vi "retrieve.vi"(8 "error in (no error)":errorcluster, 11 "DL090215DataCollection in":refnum<class "DataCollectionDL090215.lvclass">) -> (0 "error out":errorcluster, 3 "DL090215DataCollection out":refnum<class "DataCollectionDL090215.lvclass">)   [LabVIEW 2010]
uses:
  DataRequest/GenericDataRequest/GenericDataRequest/GenericDataRequest.lvclass
  common/classes/ImageCollection/ImageCollection/ImageCollection.lvclass
  common/classes/Image/Image/Image.lvclass
  common/classes/Image/Image/storage_mode.ctl
  Display/GenericDisplay/GenericDisplay/GenericDisplay.lvclass
  common/classes/ImageCollection/ImageCollection/add_mode_enum.ctl
  common/classes/ErrorController/ErrorController/ErrorController.lvclass
  DataCollectionDL090215.lvclass
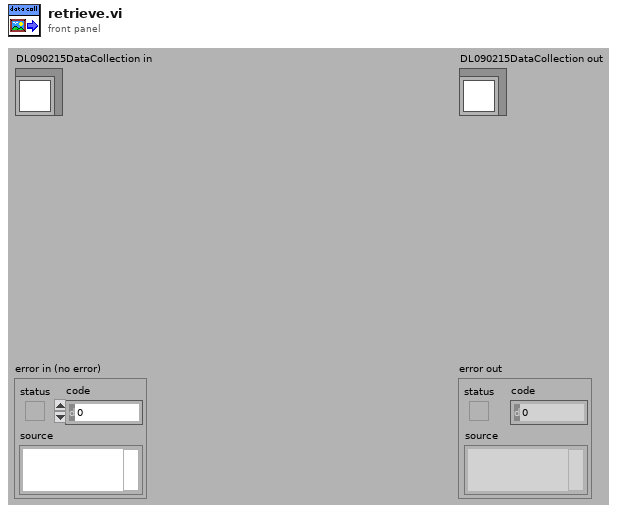
[diagram p1: front panel]
types:
  T1 = typedef "ImageCollection.lvclass/add_mode_enum.ctl" = enum16{"instance", "copy"}
  T2 = typedef "Image.lvclass/storage_mode.ctl" = enum16{"RAM", "disk"}
  T3 = typedef "GenericDataRequest.lvclass/requestor.ctl" = enum16{"NULL", "display", "analyser"}
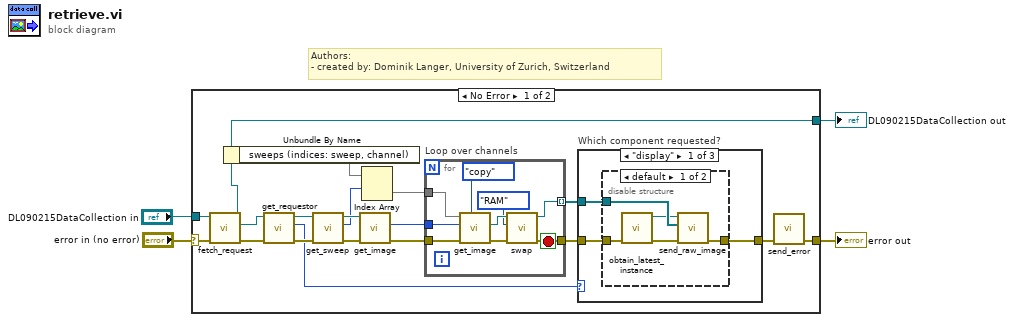
[diagram p0: block diagram]
diagram:
  # "Authors: \n- created by: Dominik Langer, University of Zurich, Switzerland"
  n1 = case shown="No Error" "error in (no error)" {
    selector: "error in (no error)" -> [w16 w45]
    tunnel: [w6 w45] -> w3
    tunnel: [w14 w44] -> w1
    tunnel: "DL090215DataCollection in" -> [w15 w44]
    frame No Error {
      n2 = call-dynamic "fetch_request.vi"("error in (no error)"=w16, "GenericDataCollection in"=w15) -> ("error out"=w11:errorcluster, "request"=w10:refnum<class "GenericDataRequest.lvclass">, "GenericDataCollection out"=w14:refnum<class "DataCollectionDL090215.lvclass">)  [unwired: 7 out]
      n3 = Unbundle By Name(w14) -> ("sweeps (indices: sweep, channel)"=w21)
      n4 = call-dynamic "get_requestor.vi"("error in (no error)"=w11, "GenericDataRequest.lvclass in"=w10) -> ("error out"=w13:errorcluster, "requestor"=w7:T3, "GenericDataRequest.lvclass out"=w12:refnum<class "GenericDataRequest.lvclass">)  [unwired: 7 out]
      n5 = call-dynamic "get_sweep.vi"("error in (no error)"=w13, "GenericDataRequest.lvclass in"=w12) -> ("error out"=w23:errorcluster, "sweep"=w20:i32, "GenericDataRequest.lvclass out"=w22:refnum<class "GenericDataRequest.lvclass">)  [unwired: 7 out]
      n6 = call-dynamic "get_image.vi"("error in (no error)"=w23, "GenericDataRequest.lvclass in"=w22) -> ("error out"=w17:errorcluster, "image"=w18:i32)  [unwired: 8 out]
      n7 = Index Array(array=w21, index (row)=w20) -> (element=w19)  [unwired: 1 in]
      n8 = for "Loop over channels" {
        tunnel: w19 -> [w42]
        tunnel: w18 -> [w41]
        tunnel: [w38] -> w8 mode=indexing
        tunnel: w17 -> [w43]
        tunnel: [w35] -> w9
        stop <- w35 stop-if-true
        n9 = call-dynamic "get_image.vi"("get image as..."=add_mode_enum."copy", "error in (no error)"=w43, "index"=w41, "ImageCollection in"=w42) -> ("error out"=w40:errorcluster, "Image.lvclass"=w39:refnum<class "Image.lvclass">)  [unwired: 6 out]
        n10 = call-dynamic "swap.vi"("error in (no error)"=w40, "storage type target"=storage_mode."RAM", "Image in"=w39) -> ("error out"=w35:errorcluster, "Image out"=w38:refnum<class "Image.lvclass">)  [unwired: 7 out]
      }
      n11 = case "Which component requested?" shown="\"display\"" w7 {
        tunnel: w9 -> [w26 w33 w34]
        tunnel: [w25 w33 w34] -> w5
        tunnel: w8 -> [w24 _ _]
        frame "display" {
          n12 = disable-structure shown="default" {
            disable-tunnel: w26 -> [w29 w32]
            disable-tunnel: [w31 w32] -> w25
            disable-tunnel: w24 -> [w30 _]
            frame condition #0 (active) {
              n13 = call "obtain_latest_instance.vi"("error in (no error)"=w29) -> ("error out"=w28:errorcluster, "GenericDisplay out"=w27:refnum<class "GenericDisplay.lvclass">)  [unwired: 1 in, 8 out]
              n14 = call-dynamic "send_raw_image.vi"("error in (no error)"=w28, "image (channels)"=w30, "GenericDisplay in"=w27) -> ("error out"=w31:errorcluster)  [unwired: 6 in, 2 out]
            }
            frame condition #1 {
            }
          }
        }
        frame "analyser" {
        }
        frame "NULL", Default {
        }
      }
      n15 = call "send_error.vi"("error in (no error)"=w5) -> ("error out"=w6:errorcluster)  [unwired: 10 in]
    }
    frame Error {
    }
  }
  "error out" <- w3
  "DL090215DataCollection out" <- w1
